vi "Xeryon Arange Parameters.vi"(6 "Parameters in":T1[](array[typedef]), 7 "Values in":i32[](array[numeric]), 9 "New drive letters":string[](array[string]), 10 "Data in":T2(array[cluster]), 11 "Known drive letters":string[](array[string])) -> (2 "Data out":T2(array[cluster]), 3 "Drive letters out":string[](array[string]))   [LabVIEW 2019]
uses:
  Class/Controller/Serial parameters.ctl
  Class/Controller/Controller.lvclass
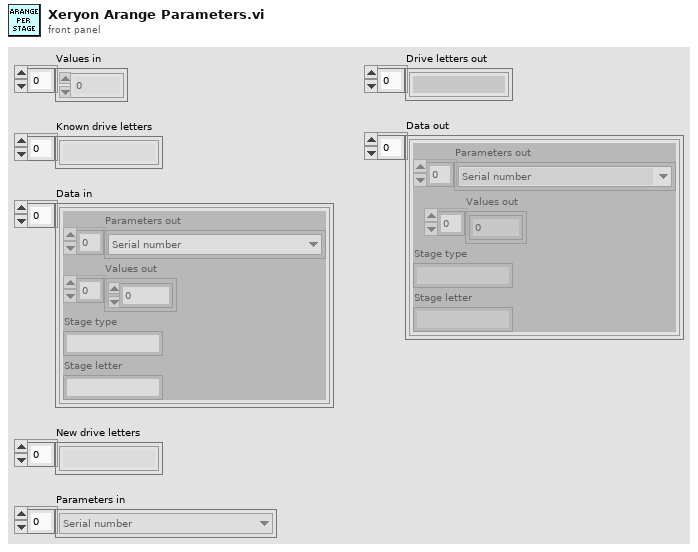
[diagram p1: front panel]
types:
  T1 = typedef "Controller.lvclass/Serial parameters.ctl" = enum16{"Serial number", "Software number", "Type of stage", "Status", "Frequency", "Encoder position", "Desired position", "Info", "Phase correction", "Timestamp", "Proportional control factor", "Sync", "XRT1", "XRT3", "XRTA", "XLS1", "XLS3", "XLA1", "XLA3"}
  T2 = cluster{"Parameters out":T1[], "Values out":i32[], "Stage type":string, "Stage letter":string}[]
  T3 = cluster{"Parameters out":T1[], "Values out":i32[], "Stage type":string, "Stage letter":string}
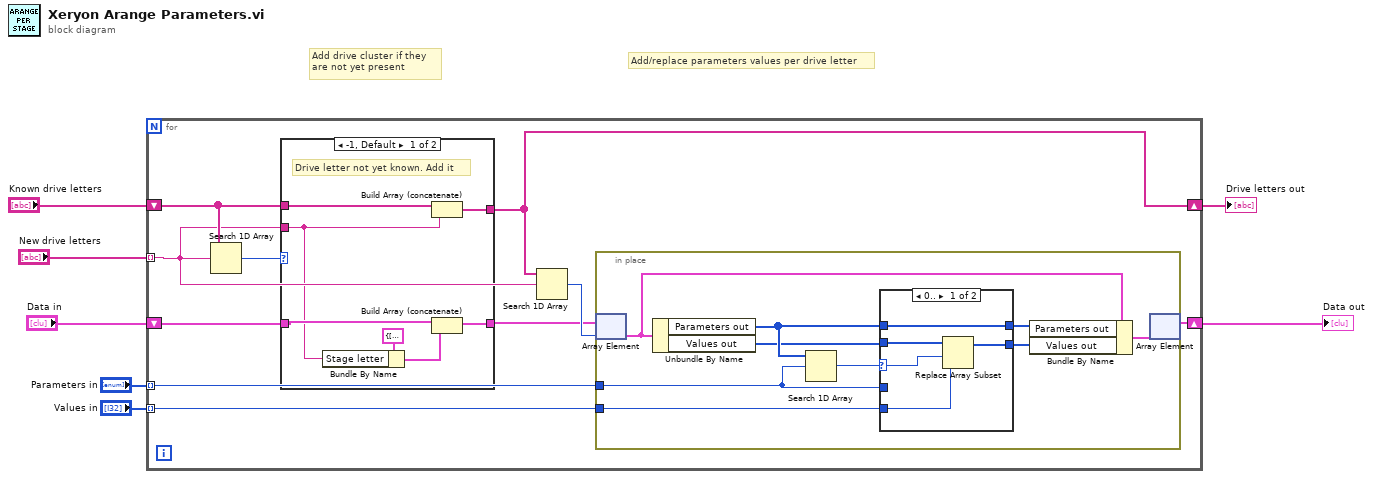
[diagram p0: block diagram]
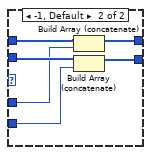
[diagram p2: hidden frame]
diagram:
  # "Add/replace parameters values per drive letter"
  # "Add drive cluster if they \nare not yet present"
  n1 = for {
    shift-right: [w9] -> w7
    shift-left: "Known drive letters" -> [w16]
    tunnel: "New drive letters" -> [w8] mode=indexing
    shift-right: [w10] -> w6
    shift-left: "Data in" -> [w15]
    tunnel: "Parameters in" -> [w12] mode=indexing
    tunnel: "Values in" -> [w11] mode=indexing
    n2 = Search 1D Array(1D array=w16, element=w8) -> (index of element=w17:i32)  [unwired: 1 in]
    n3 = case shown="-1, Default" w17 {
      tunnel: w16 -> [w44 w46]
      tunnel: w8 -> [w40 _]
      tunnel: [w43 w46] -> w9
      tunnel: w15 -> [w42 w45]
      tunnel: [w38 w45] -> w13
      frame -1, Default {
        # "Drive letter not yet known. Add it"
        n4 = Bundle By Name(cluster=T3 {"Parameters out"=[], "Values out"=[], "Stage type"="", "Stage letter"=""} ("Stage data 2"), "Stage letter"=w40) -> (w39:T3)
        n5 = Build Array (concatenate)(w44, w40) -> (w43:string[])
        n6 = Build Array (concatenate)(w42, w39) -> (w38:T2)
      }
      frame 0.. {
        # "Drive letter already present"
      }
    }
    n7 = Search 1D Array(1D array=w9, element=w8) -> (index of element=w14:i32)  [unwired: 1 in]
    n8 = in-place {
      in-place-border: w12 -> [w24]
      in-place-border: w11 -> [w22]
      n9 = in-place-array #1(w13, w14) -> (w21:T3)
      n10 = Unbundle By Name(w21) -> ("Parameters out"=w25:T1[], "Values out"=w23:i32[])
      n11 = Search 1D Array(1D array=w25, element=w24) -> (index of element=w26:i32)  [unwired: 1 in]
      n12 = case shown="0.." w26 {
        selector: w26 -> [w29 _]
        tunnel: [w31 w36] -> w20
        tunnel: w25 -> [w31 w37]
        tunnel: w23 -> [w30 w35]
        tunnel: w22 -> [w28 w33]
        tunnel: [w27 w34] -> w19
        tunnel: w24 -> [_ w32]
        frame 0.. {
          n13 = Replace Array Subset(array=w30, new element=w28, index=w29) -> (w27:i32[])
        }
        frame -1, Default {
          n14 = Build Array (concatenate)(w37, w32) -> (w36:T1[])
          n15 = Build Array (concatenate)(w35, w33) -> (w34:i32[])
        }
      }
      n16 = Bundle By Name(cluster=w21, "Parameters out"=w20, "Values out"=w19) -> (w18:T3)
      n17 = in-place-array #1(w18) -> (w10:T2)  [unwired: 1 out]
    }
  }
  "Drive letters out" <- w7
  "Data out" <- w6
